vi "Conver SNAFU Digit to Decimal number.vi"(11 "SNAFU IDs":T1) -> (3 "Decemal":i64)   [LabVIEW 2020]
uses:
  ENUM_SNAFU Digit.ctl
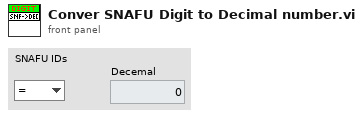
[diagram p1: front panel]
types:
  T1 = typedef "ENUM_SNAFU Digit.ctl" = enum16{"=", "-", "0", "1", "2"}
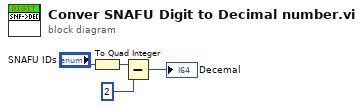
[diagram p0: block diagram]
diagram:
  n1 = To Quad Integer(1:"SNAFU IDs") -> (0:w3:i64)
  n2 = Subtract(x=w3, y=i64 2) -> (x-y=→"Decemal":i64)
